vi "PBI_MFA_Interface_DriveEnable1.vi"() -> (0 "DriveEnableStatus":bool, 1 "DriveEnableError":bool, 2 "DoCancleError":bool, 3 "BurnInError":bool)   [LabVIEW 2018]
panel:
  out "error DoCancle":errorcluster
  out "error DriveEnableOut":errorcluster
  out "error DriveEnableIn":errorcluster
  out "error BurnIn":errorcluster
  out "AAABuild":i32
  in  "MintController":refnum<k7>(container)
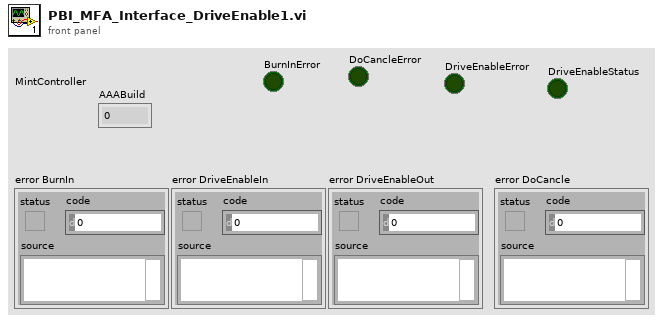
[diagram p1: front panel]
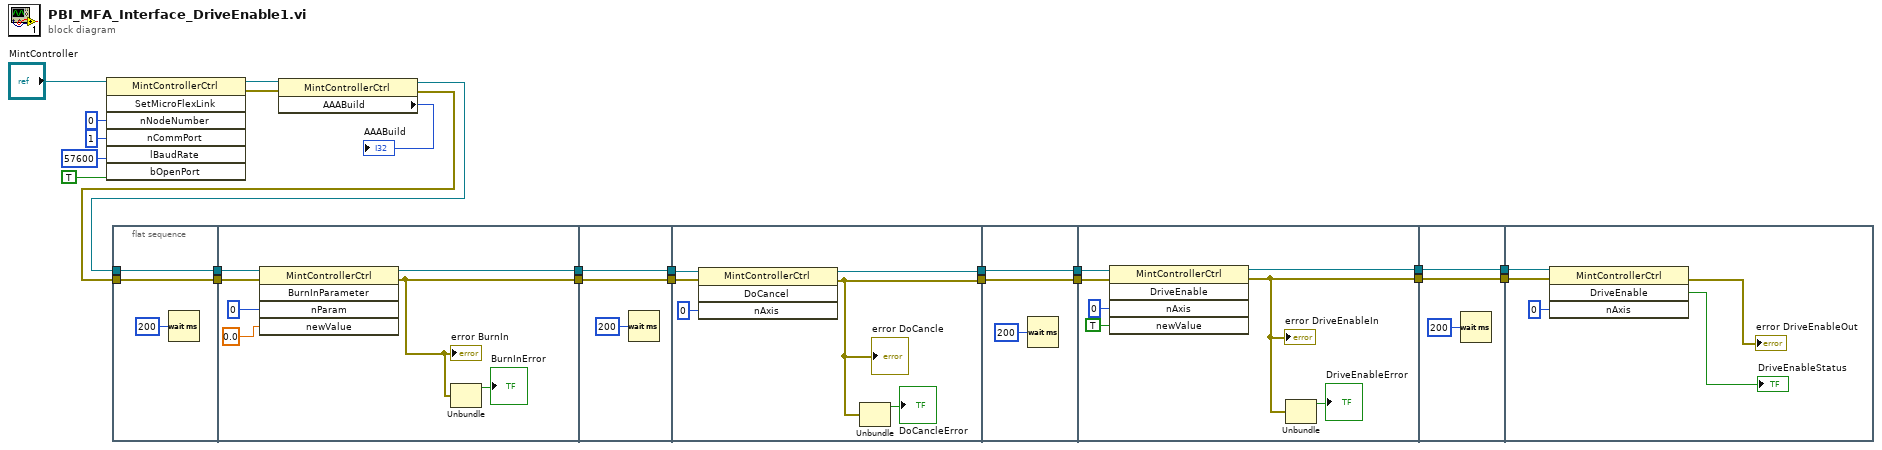
[diagram p0: block diagram]
diagram:
  n1 = invoke class="MintControllerCtrl" method="SetMicroFlexLink"(reference="MintController", "nNodeNumber"=i16 0, "nCommPort"=i16 1, "lBaudRate"=57600, "bOpenPort"=TRUE) -> (reference out=w24:refnum<k7>, error out=w18:errorcluster)  [unwired: 2 in, 5 out]
  n2 = flat-sequence {
    tunnel: [w25] -> w16
    tunnel: [w26] -> w15
    tunnel: w8 -> [w26]
    tunnel: w7 -> [w25]
    tunnel: w16 -> [w33]
    tunnel: w15 -> [w34]
    tunnel: [w29] -> w14
    tunnel: [w30] -> w13
    tunnel: w14 -> [w36]
    tunnel: w13 -> [w35]
    tunnel: [w36] -> w4
    tunnel: [w35] -> w3
    tunnel: w4 -> [w41]
    tunnel: w3 -> [w42]
    tunnel: [w43] -> w2
    tunnel: [w38] -> w1
    tunnel: [w44] -> w6
    tunnel: w2 -> [w46]
    tunnel: [w46] -> w5
    tunnel: w1 -> [w44]
    tunnel: w6 -> [w52]
    tunnel: w5 -> [w53]
    tunnel: [w47] -> w11
    tunnel: [w49] -> w9
    tunnel: [w55] -> w12
    tunnel: w11 -> [w55]
    tunnel: [w54] -> w10
    tunnel: w9 -> [w54]
    tunnel: w12 -> [w60]
    tunnel: w10 -> [w61]
    frame #0 {
      n3 = Wait (ms)(milliseconds to wait=u32 200) -> ()  [unwired: 1 out]
    }
    frame #1 {
      n4 = invoke class="MintControllerCtrl" method="BurnInParameter"(reference=w34, error in=w33, "nParam"=i16 0, "newValue"=sgl 0.0) -> (reference out=w30:refnum<k7>, error out=w29:errorcluster)  [unwired: 1 in, 3 out]
      "error BurnIn" <- w29
      n5 = Unbundle(w29) -> ("status"=→"BurnInError":bool)  [unwired: 2 out]
    }
    frame #2 {
      n6 = Wait (ms)(milliseconds to wait=u32 200) -> ()  [unwired: 1 out]
    }
    frame #3 {
      n7 = invoke class="MintControllerCtrl" method="DoCancel"(reference=w42, error in=w41, "nAxis"=i16 0) -> (reference out=w43:refnum<k7>, error out=w38:errorcluster)  [unwired: 1 in, 2 out]
      "error DoCancle" <- w38
      n8 = Unbundle(w38) -> ("status"=→"DoCancleError":bool)  [unwired: 2 out]
    }
    frame #4 {
      n9 = Wait (ms)(milliseconds to wait=u32 200) -> ()  [unwired: 1 out]
    }
    frame #5 {
      n10 = invoke class="MintControllerCtrl" method="DriveEnable"(reference=w53, error in=w52, "nAxis"=i16 0, "newValue"=TRUE) -> (reference out=w49:refnum<k7>, error out=w47:errorcluster)  [unwired: 1 in, 3 out]
      "error DriveEnableIn" <- w47
      n11 = Unbundle(w47) -> ("status"=→"DriveEnableError":bool)  [unwired: 2 out]
    }
    frame #6 {
      n12 = Wait (ms)(milliseconds to wait=u32 200) -> ()  [unwired: 1 out]
    }
    frame #7 {
      n13 = invoke class="MintControllerCtrl" method="DriveEnable"(reference=w61, error in=w60, "nAxis"=i16 0) -> (error out=→"error DriveEnableOut":errorcluster, "DriveEnable"=→"DriveEnableStatus":bool)  [unwired: 1 in, 2 out]
    }
  }
  n14 = property class="MintControllerCtrl"(reference=w24, error in=w18) -> (reference out=w8:refnum<k7>, error out=w7:errorcluster, "AAABuild"=→"AAABuild":i32)
